vi "UDP通讯.vi"() -> ()   [LabVIEW 2014]
panel:
  out "数组 2":u8[](array[numeric])
  in  "通道数光谱数据":string
  in  "发送":bool
  out "通道光谱数据图":cluster{ext[unit], ext[unit], i32[]}(graph)
  out "通道强度值数组":u8[](array[numeric])
  out "通道光谱数据":string
  out "通道6波长数值":ext[unit] format="%.2f"
  out "数组":u8[](array[numeric])
  in  "剩余量":u32
  in  "偏移量":u32
  out "通道6字符串":string
  in  "清除文本":bool
  in  "接受模式":bool
  in  "电源开关":bool
  in  "发送超时":i32
  in  "接收超时":i32
  in  "接受最大字节数":i32
  out "接收":bool
  out "接收窗口":string
  out "发送":bool
  in  "发送窗口":string
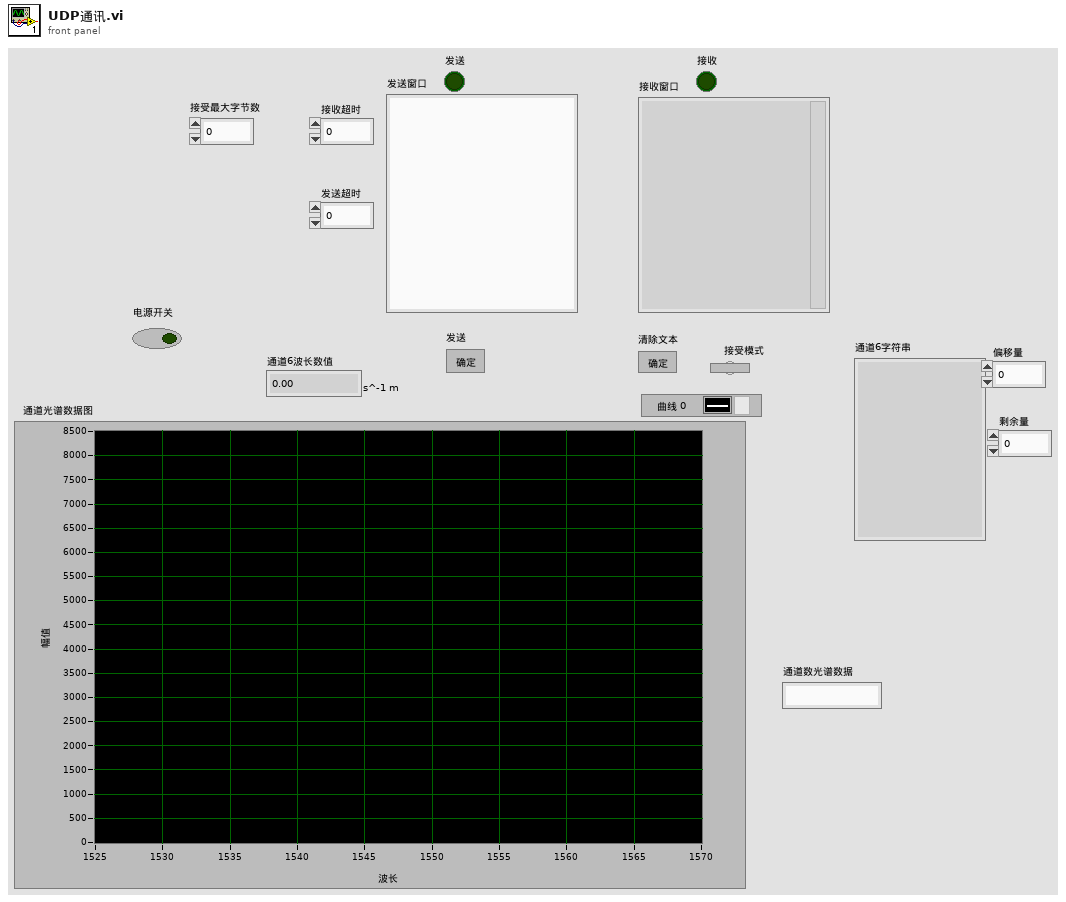
[diagram p1: front panel]
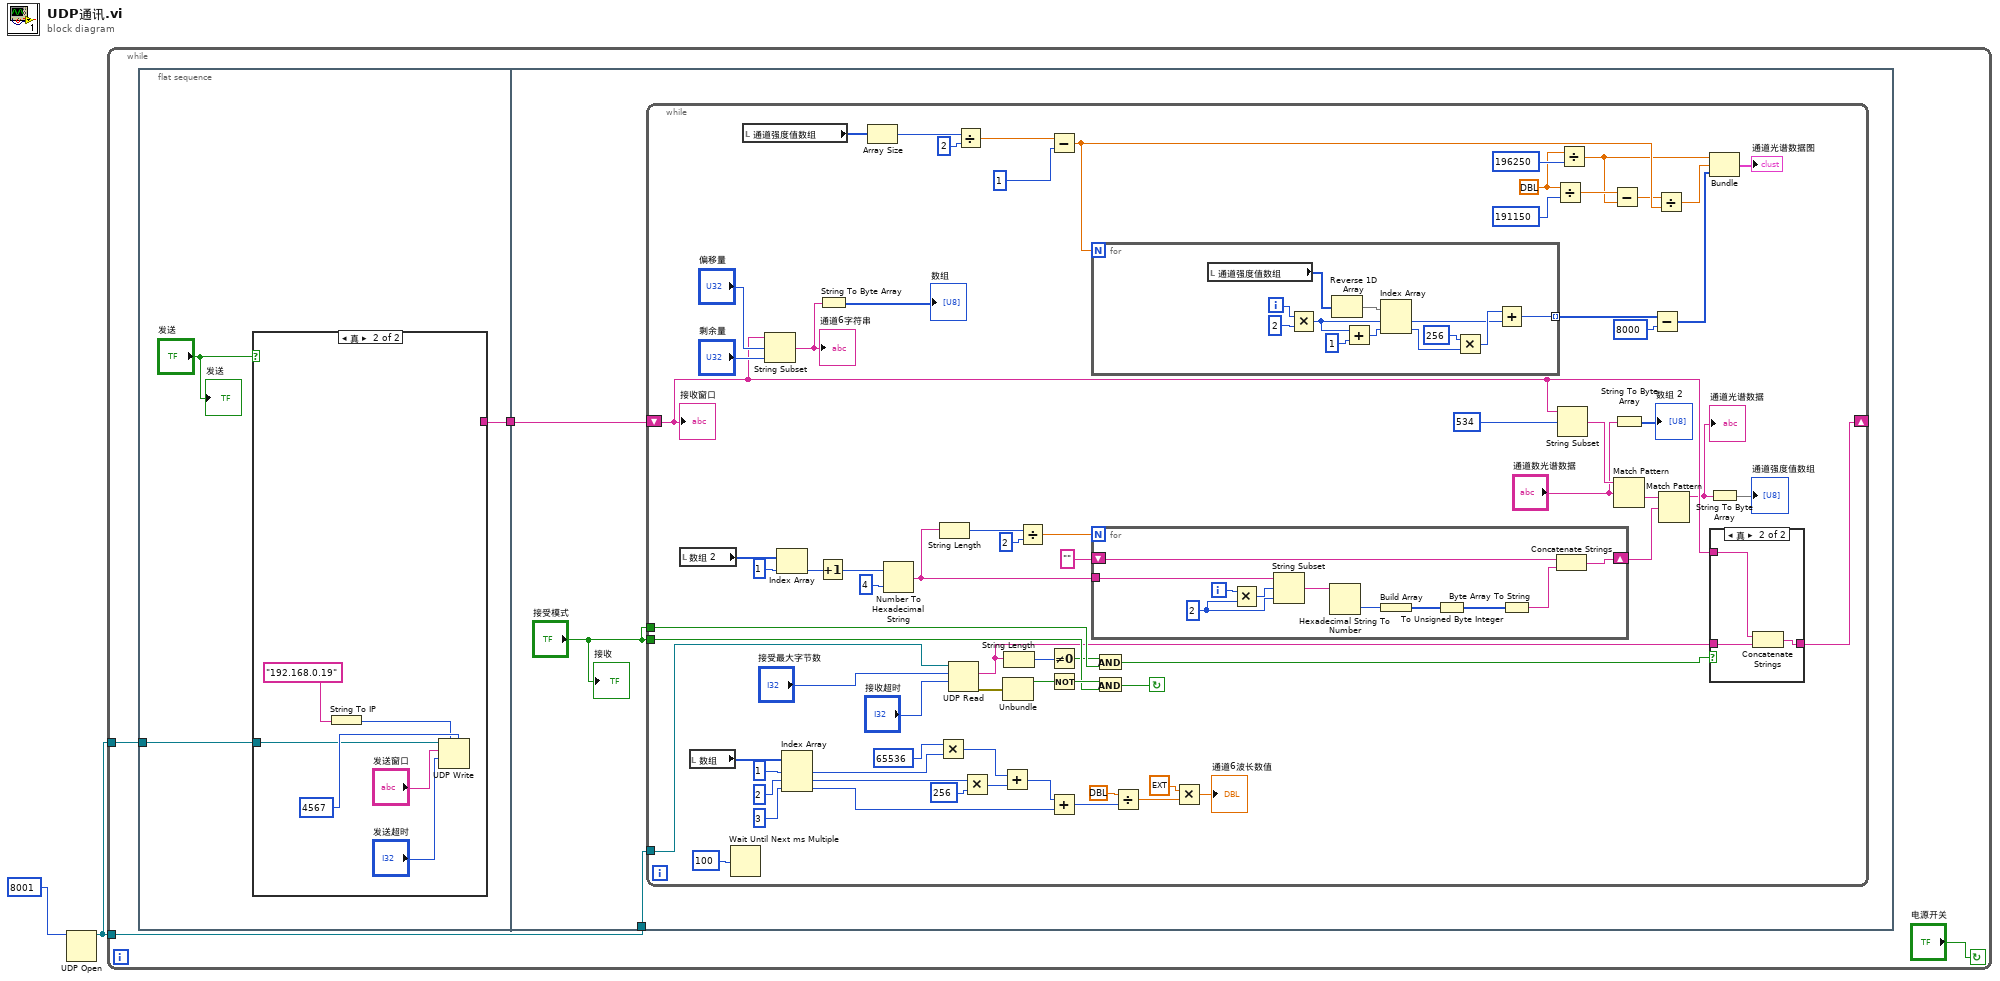
[diagram p0: block diagram]
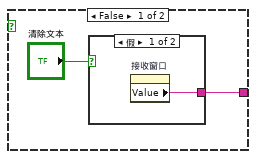
[diagram p2: hidden frame]
diagram:
  n1 = UDP Open(11:u16 8001 ("主机端口")) -> (port=w1:refnum<k16>)  [unwired: 4 in, 2 out]
  n2 = while {
    tunnel: w1 -> [w5]
    tunnel: w1 -> [w4]
    stop <- "电源开关" continue-if-true
    n3 = flat-sequence {
      tunnel: w4 -> [w8]
      tunnel: [w7] -> w3
      tunnel: w3 -> [w19]
      tunnel: w5 -> [w21]
      frame #0 {
        n4 = case shown="真" "发送" {
          tunnel: w8 -> [_ w15]
          tunnel: [w10 _] -> w7
          frame False {
            n5 = case shown="假" "清除文本" {
              tunnel: [w12 _] -> w10
              frame False {
                n6 = property on="接收窗口" class="Str"() -> ("Value"=w12:string)  [unwired: 2 in, 2 out]
              }
              frame True {
              }
            }
          }
          frame True {
            n7 = String To IP(1:"192.168.0.19" ("IP")) -> (0:w13:u32)
            n8 = UDP Write(address=w13, port or service name=u16 4567 ("客户机端口"), connection ID=w15, data in="发送窗口", 9:"发送超时") -> ()  [unwired: 1 in, 2 out]
          }
        }
        "发送" <- "发送"
      }
      frame #1 {
        n9 = while {
          shift-right: [w79] -> _
          shift-left: w19 -> [w62]
          tunnel: w21 -> [w93]
          tunnel: "接受模式" -> [w87]
          tunnel: "接受模式" -> [w84]
          stop <- w89 continue-if-true
          w26 = ext[unit] 299792458.0
          n10 = local read "数组 2"() -> (w35:u8[])
          n11 = local read "数组"() -> (w75:u8[])
          n12 = Wait Until Next ms Multiple(millisecond multiple=u32 100) -> ()  [unwired: 1 out]
          n13 = local read "通道强度值数组"() -> (w52:u8[])
          n14 = String Subset(string=w62, offset (0)="偏移量", length (rest)="剩余量") -> (substring=w76:string)
          "通道6字符串" <- w76
          n15 = Index Array(array=w35, index=1) -> (element=w34:u8)
          n16 = Index Array(array=w75, index #1=1, index #2=2, index #3=3) -> (element #1=w68:u8, element #2=w65:u8, element #3=w64:u8)
          n17 = Increment(x=w34) -> (x+1=w43:u8)
          n18 = String To Byte Array(string=w76) -> (unsigned byte array=→"数组":u8[])
          n19 = Array Size(array=w52) -> (size(s)=w50:i32)
          n20 = Number To Hexadecimal String(1:4, 2:w43) -> (0:w38:string)
          n21 = Multiply(x=65536, y=w68) -> (x*y=w71:i32)
          n22 = String Length(string=w38) -> (length=w40:i32)
          n23 = UDP Read(connection ID=w93, max size (548)="接受最大字节数", timeout ms (25000)="接收超时") -> (data out=w80:string, error out=w90:errorcluster)  [unwired: 1 in, 3 out]
          n24 = Divide(x=w50, y=2) -> (x/y=w47:dbl)
          n25 = Multiply(x=w65, y=256) -> (x*y=w70:i32)
          n26 = Add(x=w71, y=w70) -> (x+y=w69:i32)
          n27 = Unbundle(w90) -> ("status"=w86:bool)  [unwired: 2 out]
          n28 = String Length(string=w80) -> (length=w82:i32)
          n29 = Divide(x=w40, y=2 ("length")) -> (x/y=w42:dbl)
          n30 = Subtract(x=w47, y=1 ("数值")) -> (x-y=w32:dbl)
          n31 = Not Equal To 0?(x=w82) -> (x != 0?=w83:bool)
          n32 = Not(x=w86) -> (.not. x?=w88:bool)
          n33 = Add(x=w69, y=w64) -> (x+y=w63:i32)
          n34 = for {
            N: w32 -> [_]
            tunnel: [w112] -> w30 mode=indexing
            i -> [w110]
            n35 = local read "通道强度值数组"() -> (w108:u8[])
            n36 = Multiply(x=w110, y=2) -> (x*y=w109:i32)
            n37 = Reverse 1D Array(array=w108) -> (reversed array=w107:u8[])
            n38 = Add(x=w109, y=1) -> (x+y=w116:i32)
            n39 = Index Array(array=w107, index #1=w109, index #2=w116) -> (element #1=w106:u8, element #2=w105:u8)
            n40 = Multiply(x=256, y=w105) -> (x*y=w113:i32)
            n41 = Add(x=w113, y=w106) -> (x+y=w112:i32)
          }
          n42 = for {
            N: w42 -> [_]
            tunnel: w38 -> [w103]
            shift-right: [w99] -> w37
            shift-left: "" ("String") -> [w100]
            i -> [w98]
            w94 = 2 ("length (rest)")
            n43 = Multiply(x=w98, y=w94) -> (x*y=w97:i32)
            n44 = String Subset(string=w103, offset (0)=w97, length (rest)=w94) -> (substring=w102:string)
            n45 = Hexadecimal String To Number(string=w102) -> (number=w104:u32)  [unwired: 2 in, 1 out]
            n46 = Build Array(w104) -> (w96:u32[])
            n47 = To Unsigned Byte Integer(number=w96) -> (unsigned 8bit integer=w95:u8[])
            n48 = Byte Array To String(unsigned byte array=w95) -> (string=w101:string)
            n49 = Concatenate Strings(w100, w101) -> (w99:string)
          }
          n50 = And(x=w83, y=w84) -> (x .and. y?=w85:bool)
          n51 = And(x=w88, y=w87) -> (x .and. y?=w89:bool)
          n52 = Divide(x=ext[unit] 299792458.0, y=w63) -> (x/y=w57:ext[unit])
          n53 = Multiply(x=ext 10.0, y=w57) -> (x*y=→"通道6波长数值":ext[unit])
          n54 = Divide(x=w26, y=191150) -> (x/y=w25:ext[unit])
          n55 = String Subset(string=w62, offset (0)=534 ("通道移位量")) -> (substring=w54:string)  [unwired: 1 in]
          n56 = Divide(x=w26, y=196250) -> (x/y=w24:ext[unit])
          n57 = Subtract(x=w25, y=w24) -> (x-y=w23:ext[unit])
          n58 = String To Byte Array(string="通道数光谱数据") -> (unsigned byte array=→"数组 2":u8[])
          n59 = Match Pattern(string=w54, regular expression="通道数光谱数据") -> (after substring=w53:string)  [unwired: 1 in, 3 out]
          n60 = Subtract(x=w30, y=8000) -> (x-y=w29:i32[])
          n61 = Divide(x=w23, y=w32) -> (x/y=w33:ext[unit])
          n62 = Match Pattern(string=w53, regular expression=w37) -> (before substring=w51:string)  [unwired: 1 in, 3 out]
          "通道光谱数据" <- w51
          n63 = Bundle(w24, w33, w29) -> (→"通道光谱数据图":cluster{ext[unit], ext[unit], i32[]})  [unwired: 1 in]
          n64 = String To Byte Array(string=w51) -> (unsigned byte array=→"通道强度值数组":u8[])
          n65 = case shown="真" w85 {
            tunnel: w80 -> [w117 w120]
            tunnel: w62 -> [_ w119]
            tunnel: [w117 w118] -> w79
            frame False {
            }
            frame True {
              n66 = Concatenate Strings(w119, w120) -> (w118:string)
            }
          }
          "接收窗口" <- w62
        }
        "接收" <- "接受模式"
      }
    }
  }
